vi "New Figure Object.vi"(8 "error in (no error)":errorcluster) -> (0 "error out":errorcluster, 3 "Figure out":refnum<class "Figure.lvclass">)   [LabVIEW 2017, in "Styles.lvlib" / "Figure.lvclass"]
uses:
  Figure.lvclass
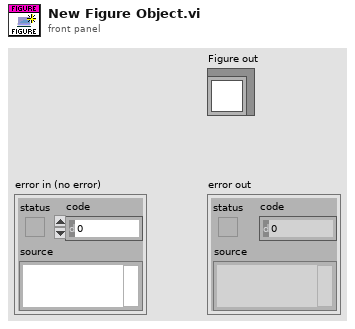
[diagram p1: front panel]
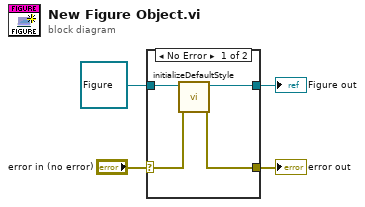
[diagram p0: block diagram]
diagram:
  n1 = case shown="No Error" "error in (no error)" {
    selector: "error in (no error)" -> [w6 w10]
    tunnel: [w5 w10] -> w3
    tunnel: [w7 w9] -> w1
    tunnel: refnum<class "Figure.lvclass"> refnum ("Figure in") -> [w8 w9]
    frame No Error {
      n2 = call-dynamic "initializeDefaultStyle.vi"("error in (no error)"=w6, "Figure in"=w8) -> ("error out"=w5:errorcluster, "Figure out"=w7:refnum<class "Figure.lvclass">)  [unwired: 8 in]
    }
    frame Error {
    }
  }
  "error out" <- w3
  "Figure out" <- w1
